vi "onProcessStopped.vi"(8 "error in (no error)":errorcluster, 11 "DAQmx-AI":refnum<class "DAQmx-AI.lvclass">) -> (0 "error out":errorcluster, 3 "DAQmx-AI out":refnum<class "DAQmx-AI.lvclass">)   [LabVIEW 2016, in "DAQmx-AI.lvclass"]
doc: "JKI State Machine Objects (SMO) 1.1.8.32\nJKI - JKI\nCopyright (c) 2016, JKI"
uses:
  DAQmx-AI.lvclass
  <vilib>/JKI/JKI SMO/SMO/SMO.lvclass
panel:
  # "For instructions on how to use the JKI State Machine Objects, examples and video tutorials, visit:\nhttp://jki.net/state-machine-objects/\n\nJKI State Machine Objects™\nhttp://jki.net/state-machine-objects/\nCopyright (C) 2005-2015, JKI <info@jki.net>\nALL RIGHTS RESERVED"
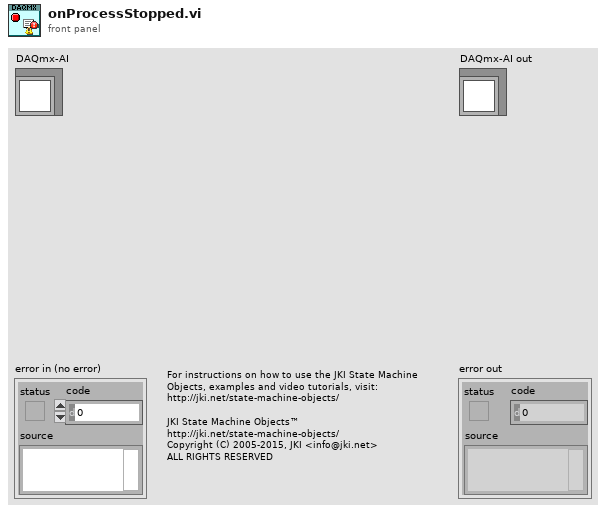
[diagram p1: front panel]
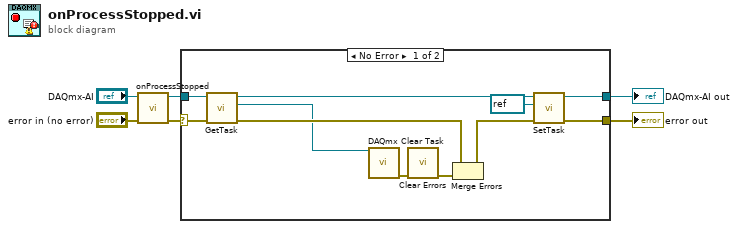
[diagram p0: block diagram]
diagram:
  n1 = call-parent "onProcessStopped.vi"("error in (no error)"="error in (no error)", "SMO"="DAQmx-AI") -> ("error out"=w4:errorcluster, "SMO out"=w3:refnum<class "DAQmx-AI.lvclass">)  [unwired: 8 in]
  n2 = case shown="No Error" w4 {
    selector: w4 -> [w16 w19]
    tunnel: w3 -> [w17 w18]
    tunnel: [w12 w18] -> w2
    tunnel: [w11 w19] -> w1
    frame No Error {
      n3 = call "GetTask.vi"("error in (no error)"=w16, "DAQmx-AI"=w17) -> ("error out"=w13:errorcluster, "task"=w7:refnum<k21>, "DAQmx-AI out"=w10:refnum<class "DAQmx-AI.lvclass">)  [unwired: 7 in]
      n4 = call <vilib>:"DAQmx Clear Task.vi"("task in"=w7) -> ("error out"=w15:errorcluster)  [unwired: 14 in]
      n5 = call <vilib>:"Clear Errors.vi"("error in (no error)"=w15) -> ("error out"=w14:errorcluster)  [unwired: 5 in, 1 out]
      n6 = Merge Errors(w13, w14) -> (w9:errorcluster)
      n7 = call "SetTask.vi"("error in (no error)"=w9, "task"=refnum<k21> refnum, "DAQmx-AI"=w10) -> ("error out"=w11:errorcluster, "DAQmx-AI out"=w12:refnum<class "DAQmx-AI.lvclass">)  [unwired: 7 in]
    }
    frame Error {
    }
  }
  "error out" <- w1
  "DAQmx-AI out" <- w2
